vi "LabVIEW Fonts.vi"(11 "Font":string) -> (3 "Desired font":T1(ring), 5 "Additional Fonts":string[](array[string]))   [LabVIEW 2021, in "lv_icon.lvlib"]
doc: "List of all LabVIEW Fonts."
uses:
  lv_icon.lvlib
panel:
  in  "String 3":string="LabVIEW Dialog"
  in  "String 2":string="LabVIEW System"
  in  "String":string="LabVIEW Application"
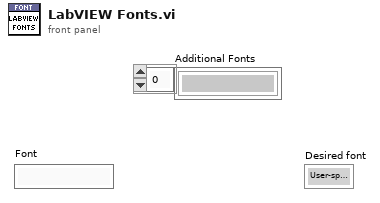
[diagram p1: front panel]
types:
  T1 = enum16{"User-specified Font", "Application Font", "System Font", "Dialog Font"}
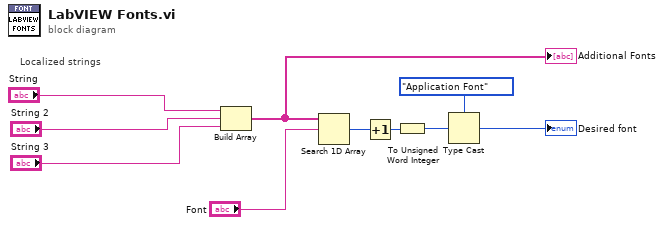
[diagram p0: block diagram]
diagram:
  # "Localized strings"
  n1 = Build Array("String", "String 2", "String 3") -> (w7:string[])
  "Additional Fonts" <- w7
  n2 = Search 1D Array(1D array=w7, element="Font") -> (index of element=w5:i32)  [unwired: 1 out]
  n3 = Increment(x=w5) -> (x+1=w4:i32)
  n4 = To Unsigned Word Integer(number=w4) -> (unsigned 16bit integer=w3:u16)
  n5 = Type Cast(type=T1."Application Font" ("desired font(Application)"), x=w3) -> (*(type *) &x=→"Desired font":T1)
